vi "Analyze and plot spectrogram .vi"(3 "change window parameters ?":bool, 4 "datalog record":T2 {"sampling frequency" format="%.2f"; "2D SGL array" format="%.6f"}) -> (0 "Spectrogram Plotting Parameters":T1 {"Dt" format="%.4f"; "Df" format="%.2f"; "f0" format="%.2f"}, 1 "Spectrogram":dbl[][](array[numeric]) format="%.6f")   [LabVIEW 2022 SP3]
doc: "Scanning signals from the doppler. WITH NO DISPLAY OF DATA FROM FFT ROUTINE"
panel:
  out "Dt":dbl format="%.2f"
  out "Rindx":i32
  out "Lindx":i32
  in  "Filter Window":T3(ring)=enum."Hanning"
  out "sampling freq.":sgl=6000.0 min=0 max=100000 format="%.2f"
  out "number of scans":u32=30000 max=1000000 step=1000
  out "sampling period":sgl format="%.3e"
  out "offset":dbl format="%.3e"
  out "data window":dbl format="%.3e"
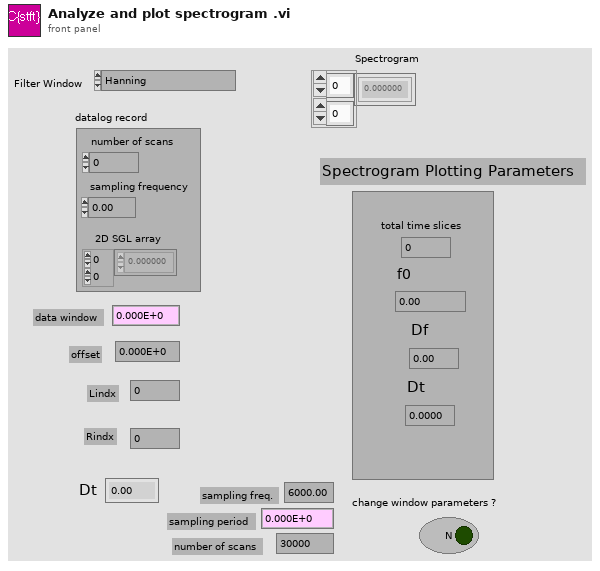
[diagram p1: front panel]
types:
  T1 = cluster{"total time slices":i32, "f0":dbl, "Df":dbl, "Dt":dbl}
  T2 = cluster{"number of scans":u32, "sampling frequency":sgl, "2D SGL array":sgl[][]}
  T3 = enum16{"None", "Hanning", "Hamming", "Triangle", "Blackman", "Exact Blackman", "Blackman-Harris", "Kaiser", "Flat Top"}
  T4 = cluster{"window width":sgl, "offset":sgl, "Lindx":i32, "Rindx":i32}
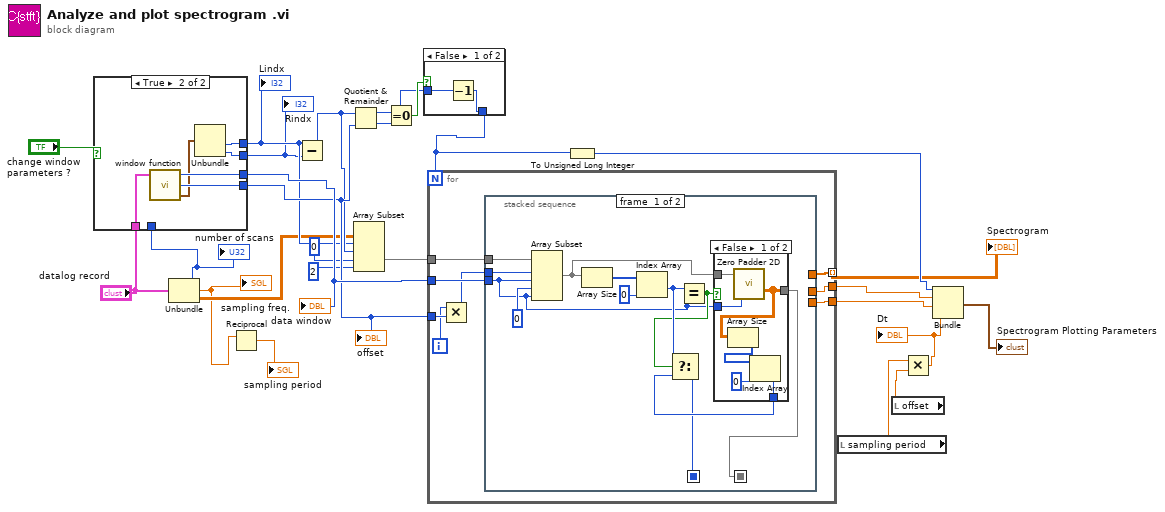
[diagram p0: block diagram]
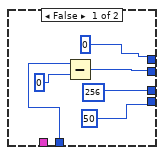
[diagram p2: hidden frame]
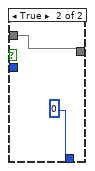
[diagram p3: hidden frame]
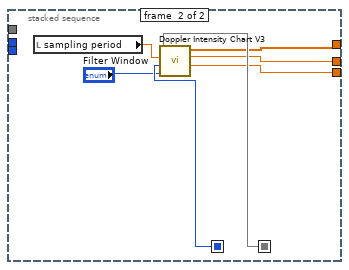
[diagram p4: hidden frame]
diagram:
  n1 = Unbundle("datalog record") -> ("number of scans"=w1:u32, "sampling frequency"=w7:sgl, "2D SGL array"=w9:sgl[][])
  "sampling freq." <- w7
  "number of scans" <- w1
  n2 = case shown="True" "change window parameters ?" {
    tunnel: [256 w38] -> w22
    tunnel: [50 w37] -> w21
    tunnel: [0 w36] -> w16
    tunnel: "datalog record" -> [_ w35]
    tunnel: [w27 w33] -> w5
    tunnel: w1 -> [w29 _]
    frame False {
      n3 = Subtract(x=w29, y=0) -> (x-y=w27:u32)
    }
    frame True {
      n4 = call "window function.vi"(5:w35) -> ("window parameters"=w34:T4, "Offset"=w37:i32, "width"=w38:i32)  [unwired: 2 in]
      n5 = Unbundle(w34) -> ("Lindx"=w36:i32, "Rindx"=w33:i32)  [unwired: 2 out]
    }
  }
  "data window" <- w22
  "offset" <- w21
  "Rindx" <- w5
  "Lindx" <- w16
  n6 = Reciprocal(x=w7) -> (1/x=→"sampling period":sgl)
  n7 = Subtract(x=w5, y=w16) -> (x-y=w17:u32)
  n8 = Quotient & Remainder(x=w17, y=w21) -> (x-y*floor(x/y)=w26:u32, floor(x/y)=w24:u32)
  n9 = Array Subset(array=w9, index (row)=w16, length (row)=w17, index (col)=0, length (col)=2) -> (w20:sgl[][])
  n10 = Equal To 0?(x=w26) -> (x = 0?=w25:bool)
  n11 = case shown="False" w25 {
    tunnel: w24 -> [w40 w41]
    tunnel: [w39 w41] -> w23
    frame False {
      n12 = Decrement(x=w40) -> (x-1=w39:u32)
    }
    frame True {
    }
  }
  n13 = for {
    N: w23 -> [_]
    tunnel: w21 -> [w49]
    tunnel: w20 -> [w46]
    tunnel: w22 -> [w48]
    tunnel: [w44] -> w3 mode=indexing
    tunnel: [w43] -> w11
    tunnel: [w42] -> w12
    i -> [w45]
    n14 = Multiply(x=w45, y=w49) -> (x*y=w47:i32)
    n15 = stacked-sequence {
      seq-local: [w54 _] -> [_ w76]
      seq-local: [w58 _] -> [_ w75]
      tunnel: w48 -> [w52 _]
      tunnel: w47 -> [w50 _]
      tunnel: w46 -> [w51 _]
      tunnel: [_ w72] -> w44
      tunnel: [_ w74] -> w43
      tunnel: [_ w73] -> w42
      frame #0 {
        n16 = Array Subset(array=w51, index (row)=w50, length (row)=w52, index (col)=0, length (col)=w52) -> (w53:sgl[][])
        n17 = Array Size(array=w53) -> (size(s)=w60:i32[])
        n18 = Index Array(array=w60, index=0) -> (element=w57:i32)
        n19 = Equal?(x=w57, y=w52) -> (x = y?=w56:bool)
        n20 = case shown="False" w56 {
          tunnel: [w66 w68] -> w58
          tunnel: w53 -> [w62 w68]
          tunnel: [w64 0] -> w55
          tunnel: w52 -> [w63 _]
          frame False {
            n21 = call "Zero Padder 2D.vi"("window size"=w63, "Input Array"=w62) -> ("Zero Padded Array"=w66:dbl[][])  [unwired: 1 in]
            n22 = Array Size(array=w66) -> (size(s)=w65:i32[])
            n23 = Index Array(array=w65, index=0) -> (element=w64:i32)
          }
          frame True {
          }
        }
        n24 = Select(t=w57, s=w56, f=w55) -> (s? t:f=w54:i32)
      }
      frame #1 {
        n25 = local read "sampling period"() -> (w71:sgl)
        n26 = call "Doppler Intensity Chart V3.vi"("Window"="Filter Window", "number of scans"=w76, "scan period"=w71, "I,Q Data"=w75) -> ("Df"=w73:dbl, "f0"=w74:dbl, "FFT Mag"=w72:dbl[])  [unwired: 2 in]
      }
    }
  }
  "Spectrogram" <- w3
  n27 = To Unsigned Long Integer(number=w23) -> (unsigned 32bit integer=w10:u32)
  n28 = local read "sampling period"() -> (w13:sgl)
  n29 = local read "offset"() -> (w14:dbl)
  n30 = Multiply(x=w13, y=w14) -> (x*y=w6:dbl)
  "Dt" <- w6
  n31 = Bundle(w10, "f0"=w11, "Df"=w12, w6) -> (→"Spectrogram Plotting Parameters":cluster{u32, "f0":dbl, "Df":dbl, dbl})  [unwired: 1 in]
